vi "LVClasse_Phase Write SurfaceFloatWithPupil.vi"(8 "error in (no error)":errorcluster, 10 "Phase":T1, 11 "Phase in":refnum<class "Phase.lvclass">) -> (0 "error out":errorcluster, 3 "Phase out":refnum<class "Phase.lvclass">)   [LabVIEW 2020, in "Phase.lvclass"]
uses:
  Phase.lvclass
  Controls/ClassID.ctl
  Controls/Handle creation.ctl
  Phase.lvclass/Phase.ctl
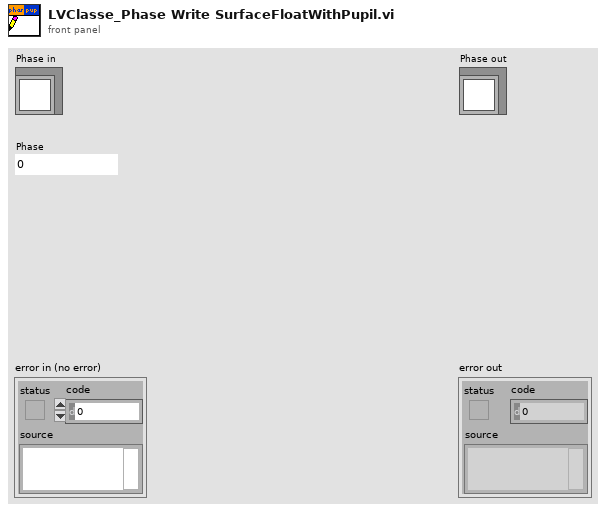
[diagram p1: front panel]
types:
  T1 = typedef "ClassID.ctl" = i64
  T2 = typedef "Handle creation.ctl" = enum16{"By ctor", "By write function"}
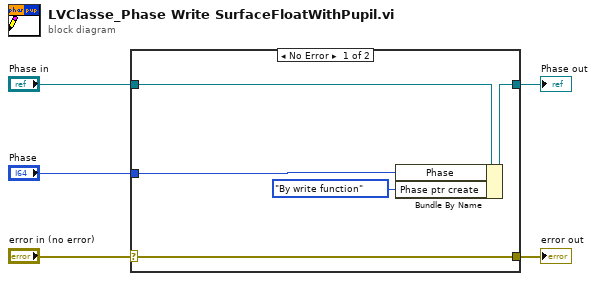
[diagram p0: block diagram]
diagram:
  n1 = case shown="No Error" "error in (no error)" {
    selector: "error in (no error)" -> [w10 w11]
    tunnel: [w10 w11] -> w4
    tunnel: [w8 w12] -> w2
    tunnel: "Phase in" -> [w9 w12]
    tunnel: "Phase" -> [w7 _]
    frame No Error {
      n2 = Bundle By Name(cluster=w9, "Phase"=w7, "Phase ptr create"=Handle_creation."By write function") -> (w8:refnum<class "Phase.lvclass">)
    }
    frame Error {
    }
  }
  "error out" <- w4
  "Phase out" <- w2
